vi "Pointer Error Info.vi"(11 "error":T1=enum."Out of Bounds") -> (3 "error info":cluster{"code":i32, "description":string})   [LabVIEW 2020, in "Memory Manager.lvlib" / "Pointer.lvclass"]
uses:
  Pointer.lvclass
  Errors.ctl
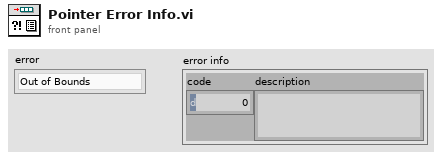
[diagram p1: front panel]
types:
  T1 = typedef "Memory Manager.lvlib/Pointer.lvclass/Errors.ctl" = enum16{"No Error", "Null Pointer", "Out of Bounds", "Buffer Underflow", "Size Mismatch", "Zone"}
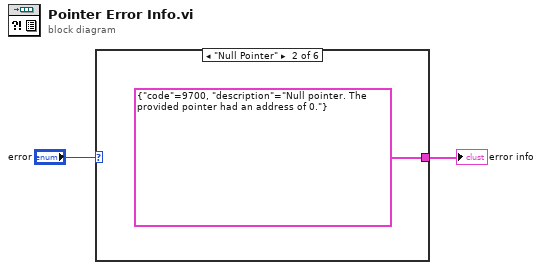
[diagram p0: block diagram]
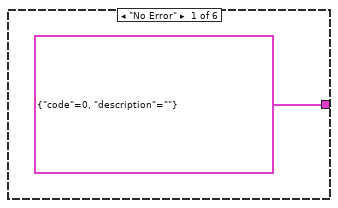
[diagram p2: hidden frame]
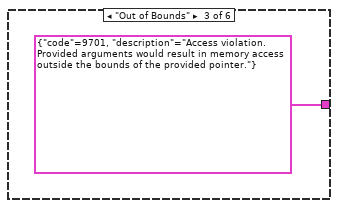
[diagram p3: hidden frame]
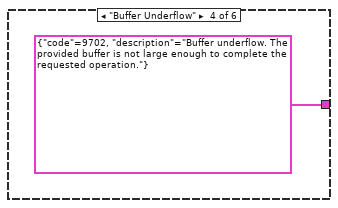
[diagram p4: hidden frame]
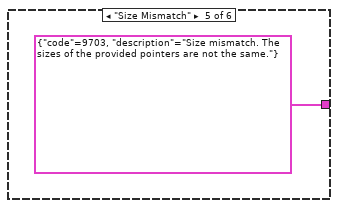
[diagram p5: hidden frame]
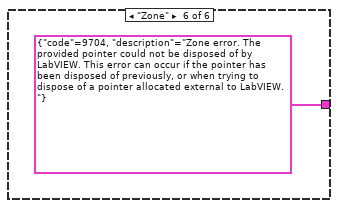
[diagram p6: hidden frame]
diagram:
  n1 = case shown="\"Null Pointer\"" "error" {
    tunnel: [cluster{"code":i32, "description":string} {"code"=0, "description"=""} ("error info") cluster{"code":i32, "description":string} {"code"=9700, "description"="Null pointer. The provided pointer had an address of 0."} ("error info") cluster{"code":i32, "description":string} {"code"=9701, "description"="Access violation. Provided arguments would result in memory access outside the bounds of the provided pointer."} ("error info") cluster{"code":i32, "description":string} {"code"=9702, "description"="Buffer underflow. The provided buffer is not large enough to complete the requested operation."} ("error info") cluster{"code":i32, "description":string} {"code"=9703, "description"="Size mismatch. The sizes of the provided pointers are not the same."} ("error info") cluster{"code":i32, "description":string} {"code"=9704, "description"="Zone error. The provided pointer could not be disposed of by LabVIEW. This error can occur if the pointer has been disposed of previously, or when trying to dispose of a pointer allocated external to LabVIEW."} ("error info")] -> w1
    frame "No Error" {
    }
    frame "Null Pointer" {
    }
    frame "Out of Bounds" {
    }
    frame "Buffer Underflow" {
    }
    frame "Size Mismatch" {
    }
    frame "Zone" {
    }
  }
  "error info" <- w1
